vi "Open Project References.vi"(8 "error in (no error)":errorcluster, 10 "Search Pattern":string, 11 "LabVIEW Build Script in":refnum<class "LabVIEW Build Script.lvclass">) -> (0 "error out":errorcluster, 3 "LabVIEW Build Script out":refnum<class "LabVIEW Build Script.lvclass">)   [LabVIEW 2021, in "LabVIEW Build Script.lvclass"]
uses:
  LabVIEW Build Script.lvclass
  LabVIEW Build Script.lvclass/LabVIEW Build Script.ctl
  <vilib>/CIF Foundation/CIF LabVIEW Scripting/LV Scripting/LV Scripting Utilities.lvlib
  Build Script Common/Typedef/Build Script Errors.ctl
  Build Script Common/Build Script Common.lvlib
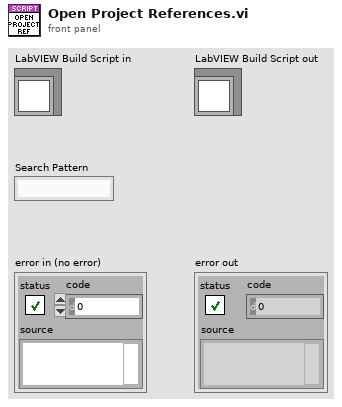
[diagram p1: front panel]
types:
  T1 = typedef "Build Script Common.lvlib/Build Script Errors.ctl" = enum16{"Item not found"}
  T2 = typedef "LV Scripting Utilities.lvlib/Target References.ctl" = cluster{"Target Reference":refnum<vi>, "VI References":refnum<vi>[], "Library References":refnum<vi>[], "Build References":refnum<vi>[]}
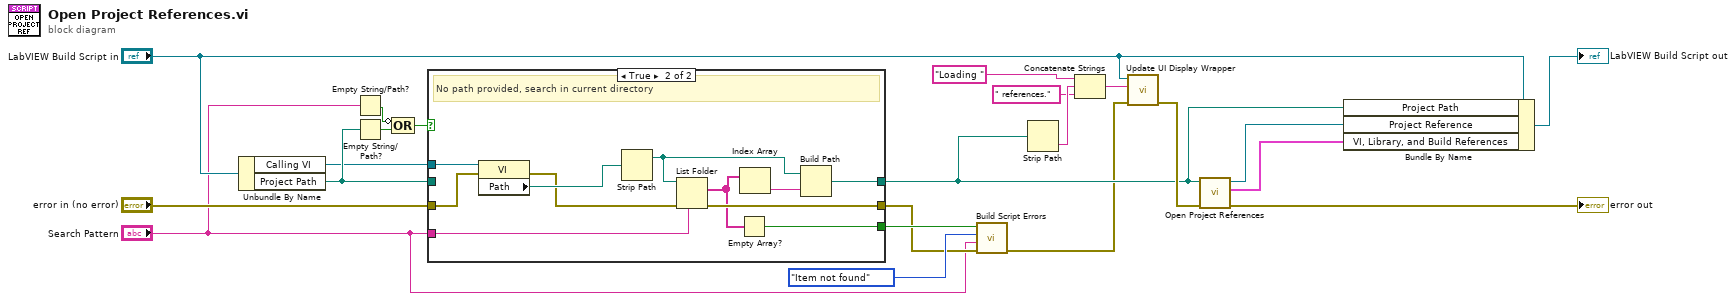
[diagram p0: block diagram]
diagram:
  n1 = Unbundle By Name("LabVIEW Build Script in") -> ("Calling VI"=w6:refnum<vi>, "Project Path"=w21:path)
  n2 = Empty String/Path?(string/path="Search Pattern") -> (empty?=w7:bool)
  n3 = Empty String/Path?(string/path=w21) -> (empty?=w9:bool)
  n4 = Compound Arithmetic op=OR(invert w7, w9) -> (w8:bool)
  n5 = case shown="True" w8 {
    tunnel: [w24 w34] -> w14
    tunnel: [w23 w33] -> w3
    tunnel: "Search Pattern" -> [_ w31]
    tunnel: w21 -> [w24 _]
    tunnel: "error in (no error)" -> [w23 w27]
    tunnel: [_ w29] -> w4
    tunnel: w6 -> [_ w28]
    frame False {
      # "Path provided"
    }
    frame True {
      # "No path provided, search in current directory"
      n6 = property class="VI"(reference=w28, error in=w27) -> (error out=w25:errorcluster, "Path"=w26:path)  [unwired: 1 out]
      n7 = Strip Path(path=w26) -> (stripped path=w32:path)  [unwired: 1 out]
      n8 = List Folder(path=w32, pattern=w31, error in=w25) -> (filenames=w30:string[], error out=w33:errorcluster)  [unwired: 1 in, 2 out]
      n9 = Empty Array?(array=w30) -> (empty?=w29:bool)
      n10 = Index Array(array=w30) -> (element=w35:string)  [unwired: 1 in]
      n11 = Build Path(base path=w32, name or relative path=w35) -> (appended path=w34:path)
    }
  }
  n12 = call "Build Script Errors.vi"("error in (no error)"=w3, "String to Append"="Search Pattern", "Error"=Build_Script_Errors."Item not found", "Insert Error"=w4) -> ("error out"=w1:errorcluster)  [unwired: 7 in]
  n13 = Strip Path(path=w14) -> (name=w17:string)  [unwired: 1 out]
  n14 = Concatenate Strings("Loading " ("Update for Display"), w17, " references." ("string")) -> (w16:string)
  n15 = call "Update UI Display Wrapper.vi"("error in (no error)"=w1, "Update for Display"=w16, "LabVIEW Build Script in"="LabVIEW Build Script in") -> ("error out"=w20:errorcluster)  [unwired: 8 in]
  n16 = call <vilib>:"Open Project References.vi"("error in"=w20, "Project Path"=w14) -> ("error out"=→"error out":errorcluster, "VI, Library, and Build References"=w12:T2[], "Project Reference"=w13:refnum<vi>)  [unwired: 7 in]
  n17 = Bundle By Name(cluster="LabVIEW Build Script in", "Project Path"=w14, "Project Reference"=w13, "VI, Library, and Build References"=w12) -> (→"LabVIEW Build Script out":refnum<class "LabVIEW Build Script.lvclass">)
